vi "Emballage_BDD_Update_SQL.vi"(5 "SN_PRODUIT ancien":string, 6 "NO_DU_CARTON":string, 7 "ID_UTILISATEUR_GPAO":string, 8 "error in (no error)":errorcluster, 9 "NO_CDEVAL":string, 10 "SN_PRODUIT":string, 11 "Table":string) -> (0 "error out":errorcluster)   [LabVIEW 2020]
uses:
  Modules/FS/60_FS_Controles/60_FS_SetGet.ctl
  <vilib>/addons/database/Connection.llb/DB Tools Open Connec (Path).vi
  <vilib>/addons/database/Connection.llb/Conn Execute.vi
  <vilib>/addons/database/Recordset.llb/Rec Destroy - Connection.vi
  <vilib>/addons/database/NI_Database_API.lvlib
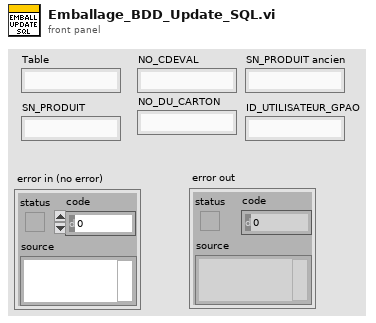
[diagram p1: front panel]
types:
  T1 = typedef "60_FS_SetGet.ctl" = enum16{"set", "get"}
  T2 = typedef "60_FS_CLT_Chemins.ctl" = cluster{"Racine_local":path, "Racine_reseau":path, "Racine_Support_Application":path, "Fichier_Journalisation":path, "Connexion_BDD_VSX":path, "Connexion_BDD_PLZ":path}
  T3 = typedef "NI_Database_API.lvlib/Conn ObjectReference.ctl" = refnum<k1>
  T4 = typedef "NI_Database_API.lvlib/Rec ObjectReference.ctl" = refnum<k1>
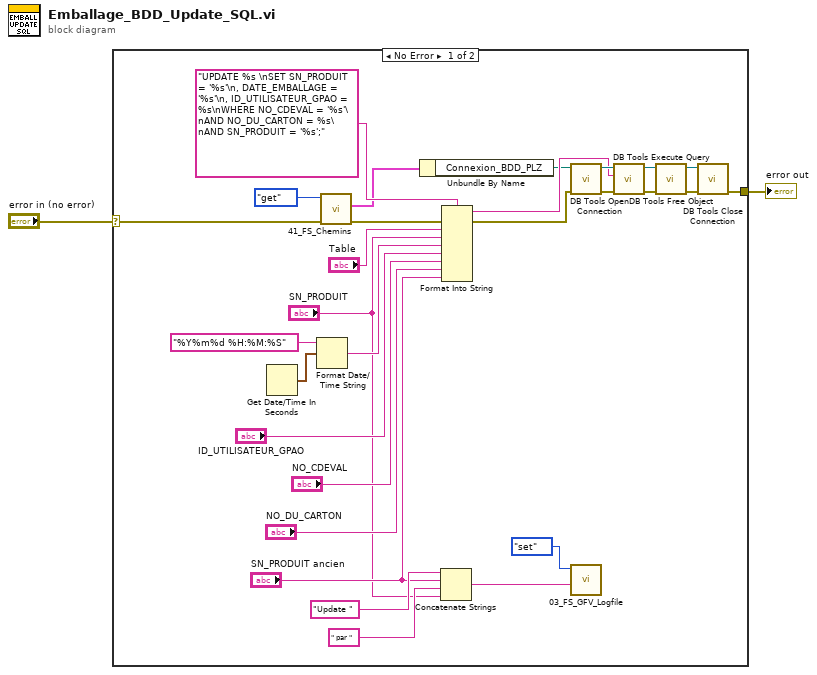
[diagram p0: block diagram]
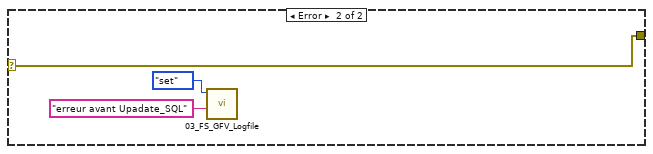
[diagram p2: hidden frame]
diagram:
  n1 = case shown="No Error" "error in (no error)" {
    selector: "error in (no error)" -> [w16 w33]
    tunnel: [w15 w33] -> w1
    frame No Error {
      n2 = Get Date/Time In Seconds() -> (seconds since 1Jan1904=w10:timestamp)
      n3 = Format Date/Time String(time format string (%c)="%Y%m%d %H:%M:%S" ("chaîne de format de l'heure (%c)"), seconds (now)=w10) -> (date/time string=w9:string)  [unwired: 1 in]
      n4 = call "41_FS_Chemins.vi"("error in (no error)"=w16, "SetGet"=60_FS_SetGet."get") -> ("error out"=w17:errorcluster, "CLT_Chemins_out"=w21:T2)  [unwired: 8 in]
      n5 = Unbundle By Name(w21) -> ("Connexion_BDD_PLZ"=w19:path)
      n6 = Concatenate Strings("Update " ("chaîne"), "SN_PRODUIT ancien", " par " ("chaîne"), "SN_PRODUIT") -> (w3:string)
      n7 = Format Into String(format string="UPDATE %s \nSET SN_PRODUIT = '%s'\n, DATE_EMBALLAGE = '%s'\n, ID_UTILISATEUR_GPAO = %s\nWHERE NO_CDEVAL = '%s'\nAND NO_DU_CARTON = %s\nAND SN_PRODUIT = '%s';" ("chaîne de format"), error in=w17, "Table", "SN_PRODUIT", w9, "ID_UTILISATEUR_GPAO", "NO_CDEVAL", "NO_DU_CARTON", "SN_PRODUIT ancien") -> (resulting string=w24:string, error out=w22:errorcluster)  [unwired: 1 in]
      n8 = call-poly <vilib>:"DB Tools Open Connection.vi"("error in (no error)"=w22, "connection information"=w19) -> ("error out"=w30:errorcluster, "connection reference"=w25:T3)  [unwired: 6 in]
      n9 = call "03_FS_GFV_Logfile.vi"("Chaîne"=w3, "States"=60_FS_SetGet."set") -> ()  [unwired: 8 in, 2 out]
      n10 = call-poly <vilib>:"DB Tools Execute Query.vi"("error in (no error)"=w30, "SQL query"=w24, "connection reference"=w25) -> ("error out"=w29:errorcluster, "recordset reference"=w28:T4)  [unwired: 5 in]
      n11 = call-poly <vilib>:"DB Tools Free Object.vi"("error in (no error)"=w29, "recordset reference"=w28) -> ("error out"=w27:errorcluster, "connection reference"=w26:T3)  [unwired: 8 in]
      n12 = call <vilib>:"DB Tools Close Connection.vi"("error in (no error)"=w27, "connection reference"=w26) -> ("error out"=w15:errorcluster)  [unwired: 5 in]
    }
    frame Error {
      n13 = call "03_FS_GFV_Logfile.vi"("Chaîne"="erreur avant Upadate_SQL", "States"=60_FS_SetGet."set") -> ()  [unwired: 8 in, 2 out]
    }
  }
  "error out" <- w1
